vi "MTS_CalcMeasTime.vi"(0 "Scanner Divider":i32, 1 "pt3 header in":T1={"Comment"="", "RangeNo"=0, "Offset"=0, "AcquisitionTime (ms)"=0, "HardwareSerial"=0, "SyncDivider"=0, "Resolution (ns)"=0.0, "CFD Settings"={"Ch0 Level"=150, "Ch0 ZeroX"=10, "Ch1 Level"=50, "Ch1 ZeroX"=10}, "InpRate0"=0, "InpRate1"=0}, 7 "Measurement time [s]":i32, 11 "Count Rate":i32) -> (3 "pt3 header out":T1={"Comment"="", "RangeNo"=0, "Offset"=0, "AcquisitionTime (ms)"=0, "HardwareSerial"=0, "SyncDivider"=0, "Resolution (ns)"=0.0, "CFD Settings"={"Ch0 Level"=150, "Ch0 ZeroX"=10, "Ch1 Level"=50, "Ch1 ZeroX"=10}, "InpRate0"=0, "InpRate1"=0}, 4 "Corrected Measurement time [s]":i32, 6 "Calc Acq. Time (ms)":i32, 10 "Overflow Interv. Time (s)":dbl, 15 "Pixel Time (Laser Pulses)":i32)   [LabVIEW 2010]
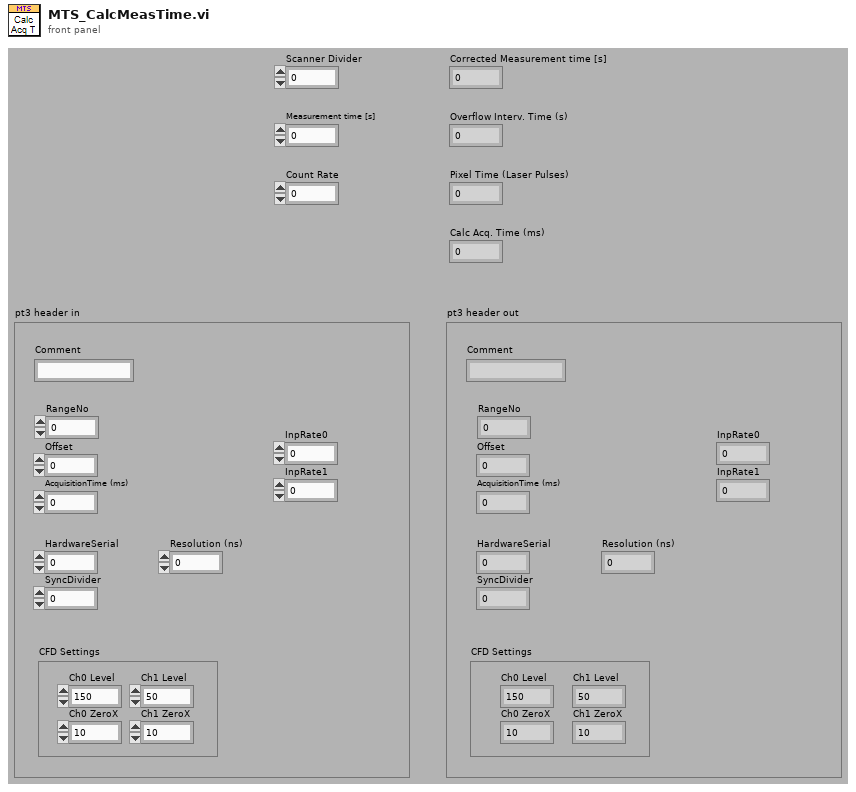
[diagram p1: front panel]
types:
  T1 = cluster{"Comment":string, "RangeNo":i32, "Offset":i32, "AcquisitionTime (ms)":i32, "HardwareSerial":i32, "SyncDivider":i32, "Resolution (ns)":sgl, "CFD Settings":cluster{"Ch0 Level":i32, "Ch0 ZeroX":i32, "Ch1 Level":i32, "Ch1 ZeroX":i32}, "InpRate0":i32, "InpRate1":i32}
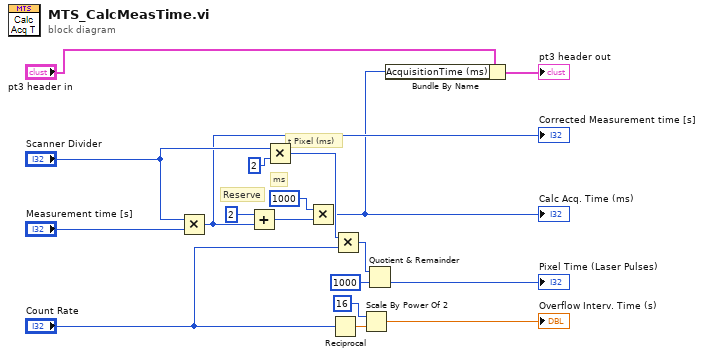
[diagram p0: block diagram]
diagram:
  # "t Pixel (ms)"
  # "ms"
  # "Reserve"
  n1 = Multiply(x="Scanner Divider", y="Measurement time [s]") -> (x*y=w5:i32)
  "Corrected Measurement time [s]" <- w5
  n2 = Add(x=2, y=w5) -> (x+y=w7:i32)
  n3 = Multiply(x="Scanner Divider", y=2 ("x")) -> (x*y=w13:i32)
  n4 = Multiply(x=1000, y=w7) -> (x*y=w2:i32)
  "Calc Acq. Time (ms)" <- w2
  n5 = Reciprocal(x="Count Rate") -> (1/x=w11:dbl)
  n6 = Multiply(x=w13, y="Count Rate") -> (x*y=w15:i32)
  n7 = Scale By Power Of 2(n=16, x=w11) -> (x*2^n=→"Overflow Interv. Time (s)":dbl)
  n8 = Quotient & Remainder(x=w15, y=1000) -> (floor(x/y)=→"Pixel Time (Laser Pulses)":i32)  [unwired: 1 out]
  n9 = Bundle By Name(cluster="pt3 header in", "AcquisitionTime (ms)"=w2) -> (→"pt3 header out":T1)
